vi "Format Log Data.vi"(8 "error in (no error)":errorcluster, 9 "Channels":waveform(dbl)[](array[waveform]), 11 "Data Logger Module in":refnum<class "Data Logger DBL Module.lvclass">) -> (0 "error out":errorcluster, 1 "Data":dbl[][](array[numeric]), 2 "Time":i64[](array[numeric]), 3 "Data Logger Module out":refnum<class "Data Logger DBL Module.lvclass">, 5 "Relative Time":dbl[](array[numeric]))   [LabVIEW 2020, in "VolatusData.lvlib" / "Data Logger DBL Module.lvclass"]
uses:
  Data Logger DBL Module.lvclass
  Data Logger DBL Module.lvclass/Data Logger DBL Module.ctl
  lv-vecto/Vecto/Vecto.lvlib
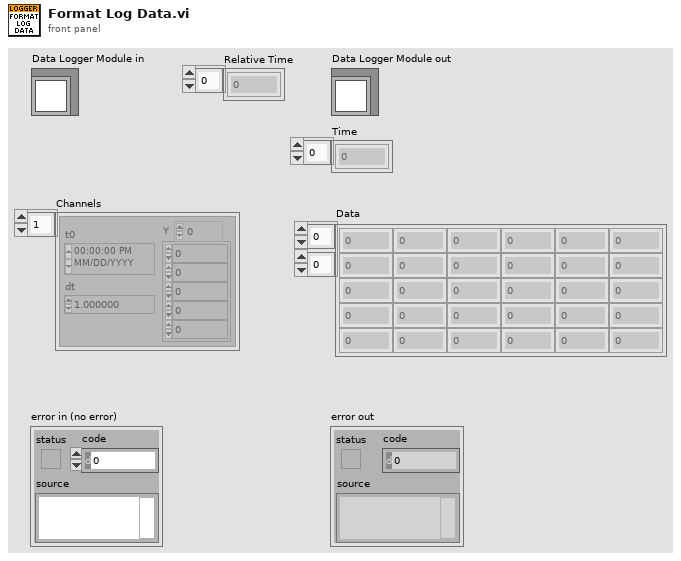
[diagram p1: front panel]
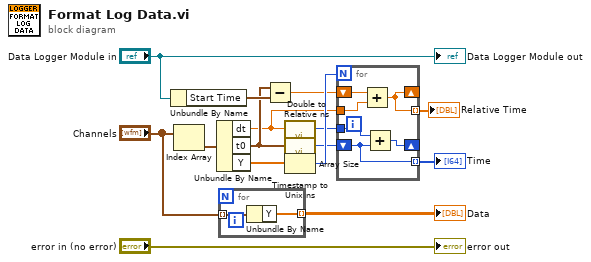
[diagram p0: block diagram]
diagram:
  n1 = Unbundle By Name("Data Logger Module in") -> ("Start Time"=w5:timestamp)
  n2 = Index Array(array="Channels") -> (element=w14:waveform(dbl))  [unwired: 1 in]
  n3 = Unbundle By Name(w14) -> ("dt"=w3:dbl, "t0"=w4:timestamp, "Y"=w13:dbl[])
  n4 = for {
    tunnel: "Channels" -> [w17] mode=indexing
    tunnel: [w16] -> w10 mode=indexing
    n5 = Unbundle By Name(w17) -> ("Y"=w16:dbl[])
  }
  "Data" <- w10
  n6 = Subtract(x=w4, y=w5) -> (x-y=w2:dbl)
  n7 = call "Double to Relative ns.vi"("Double"=w3) -> ("Relative ns"=w8:i64)  [unwired: 2 in]
  n8 = call "Timestamp to Unix ns.vi"("Time Stamp"=w4) -> ("unix ns"=w9:i64)  [unwired: 2 in]
  n9 = Array Size(array=w13) -> (size(s)=w12:i32)
  n10 = for {
    N: w12 -> [_]
    shift-right: [w21] -> _
    shift-left: w9 -> [w23]
    tunnel: w8 -> [w22]
    tunnel: [w23] -> w7 mode=indexing
    tunnel: w3 -> [w19]
    shift-right: [w18] -> _
    shift-left: w2 -> [w20]
    tunnel: [w18] -> w1 mode=indexing
    (unwired) 0.0 ("x+y")
    n11 = Add(x=w20, y=w19) -> (x+y=w18:dbl)
    n12 = Add(x=w22, y=w23) -> (x+y=w21:i64)
  }
  "Time" <- w7
  "Relative Time" <- w1
  "error out" <- "error in (no error)"
  "Data Logger Module out" <- "Data Logger Module in"
